vi "Pressure Temperature Monitor v2.vi"() -> ()   [LabVIEW 2016]
panel:
  in  "?":i32(ring)=1 items=["MKS 943 Cold Cathode"=1, "Thyracont All Range"=2]
  in  "?":i32(ring)=2 items=["MKS 943 Cold Cathode"=1, "Thyracont All Range"=2]
  in  "?":bool
  out "Pressure CH2":dbl=3.6243247155441205e-08 format="%#.2e"
  out "LL Pressure":dbl(graph)=3.6243247155441205e-08
  out "Tempreture CH2":dbl=27.062558993140346 format="%.1f"
  out "T2 Tempreture":dbl(graph)=27.062558993140346
  in  "Gain":dbl=-10.0 format="%#_13g"
  in  "Gain":dbl=-11.0 format="%#_13g"
  out "Tempreture CH1":dbl=400.77454527767986 format="%.1f"
  out "Pressure CH1":dbl=1.7126957385138226e-08 format="%#.2e"
  out "Heater Tempreture":dbl(graph)=400.77454527767986
  in  "?":bool
  out "Overdosing":bool
  in  "Dosing Limit":dbl=20.0 format="%#.2f"
  in  "Base Pressure":dbl=6.47 format="%#.2e"
  out "PRE Pressure":dbl(graph)=1.7126957385138226e-08
  out "L":dbl format="%.1f"
  in  "Pressure Limit":dbl=10.0 format="%#.2e"
  in  "?":bool
  # "LL Pressure (Torr)"
  # "PRE Pressure"
  # "Langmuir"
  # "(Torr)"
  # "(Torr)"
  # "CH1"
  # "CH2"
  # "Heater Temperature"
  # "T2"
  # "(°C )"
  # "(°C )"
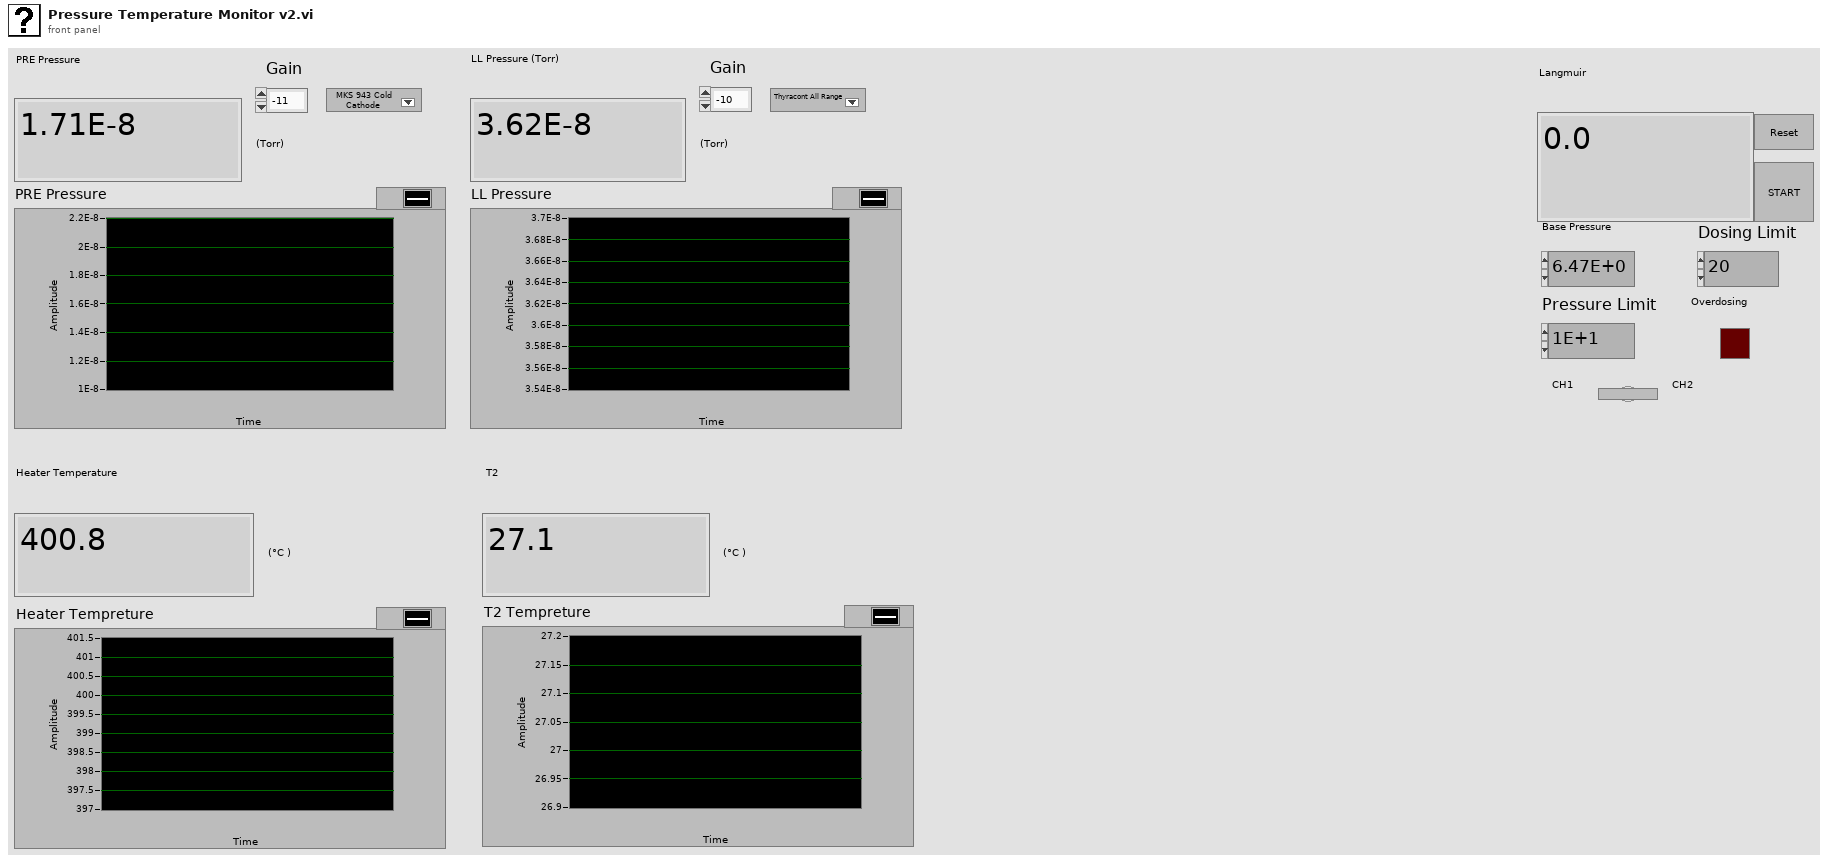
[diagram p1: front panel]
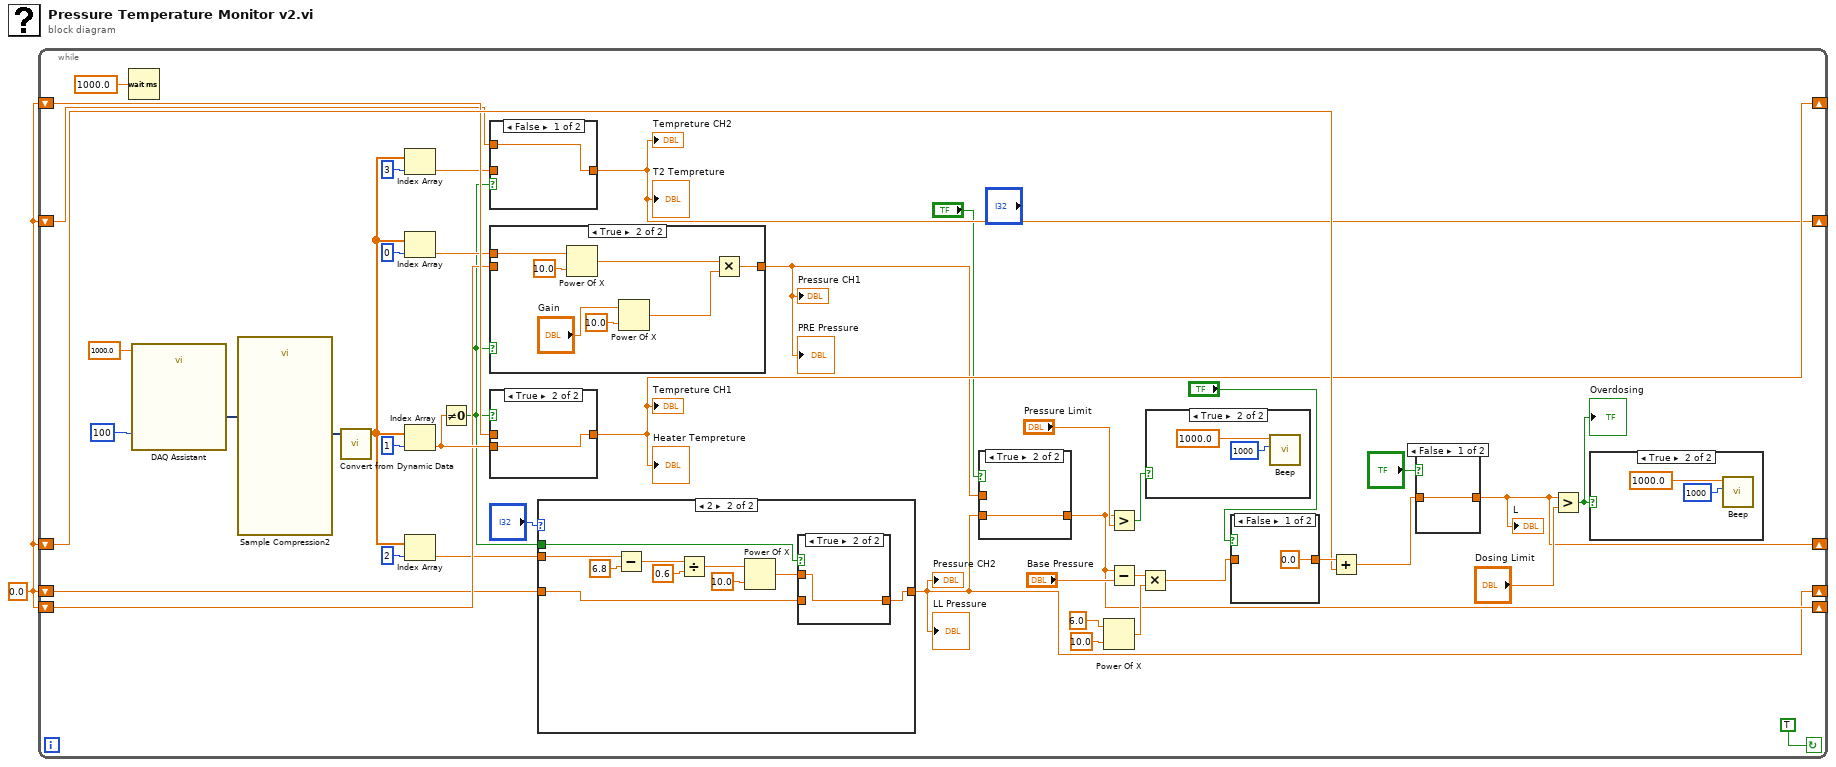
[diagram p0: block diagram]
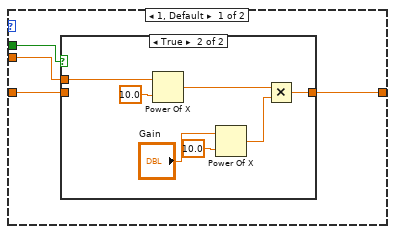
[diagram p2: hidden frame]
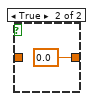
[diagram p9: hidden frame]
diagram:
  w1 = 0.0
  n1 = while {
    shift-left: w1 -> [w35]
    shift-right: [w33] -> _
    shift-right: [w6] -> _
    shift-left: w1 -> [w26]
    shift-right: [w25] -> _
    shift-left: w1 -> [w29]
    shift-right: [w4] -> _
    shift-left: w1 -> [w12]
    shift-right: [w9] -> _
    shift-left: w1 -> [w10]
    stop <- TRUE continue-if-true
    n2 = Wait (ms)(milliseconds to wait=1000.0 ("y")) -> ()  [unwired: 1 out]
    n3 = call "DAQ Assistant"("rate"=1000.0, "number of samples"=100) -> ("data"=w17:dynamicdata)  [unwired: 15 in, 2 out]
    n4 = call "Sample Compression2"("Signals"=w17) -> ("Mean"=w14:dynamicdata)  [unwired: 8 in, 2 out]
    n5 = call "Convert from Dynamic Data"("Dynamic Data Type"=w14) -> ("Array"=w3:dbl[])  [unwired: 3 in]
    n6 = Index Array(array=w3, index=3) -> (element=w11:dbl)
    n7 = Index Array(array=w3, index=0) -> (element=w27:dbl)
    n8 = Index Array(array=w3, index=1) -> (element=w28:dbl)
    n9 = Index Array(array=w3, index=2) -> (element=w13:dbl)
    n10 = Not Equal To 0?(x=w28) -> (x != 0?=w2:bool)
    n11 = case shown="False" w2 {
      tunnel: w10 -> [w71 _]
      tunnel: [w71 w72] -> w9
      tunnel: w11 -> [_ w72]
      frame False {
      }
      frame True {
      }
    }
    "T2 Tempreture" <- w9
    "Tempreture CH2" <- w9
    n12 = case shown="True" w2 {
      tunnel: w27 -> [_ w79]
      tunnel: [w73 w80] -> w7
      tunnel: w26 -> [w73 _]
      frame False {
      }
      frame True {
        n13 = Power Of X(1:10.0 ("x"), 2:w79) -> (0:w78:dbl)
        n14 = Power Of X(1:10.0 ("x"), 2:"Gain") -> (0:w76:dbl)
        n15 = Multiply(x=w78, y=w76) -> (x*y=w80:dbl)
      }
    }
    "PRE Pressure" <- w7
    "Pressure CH1" <- w7
    n16 = case shown="True" w2 {
      tunnel: w28 -> [_ w82]
      tunnel: [w81 w82] -> w25
      tunnel: w29 -> [w81 _]
      frame False {
      }
      frame True {
      }
    }
    "Heater Tempreture" <- w25
    "Tempreture CH1" <- w25
    n17 = case shown="2" "?" {
      tunnel: w2 -> [w48 w58]
      tunnel: w13 -> [w47 w57]
      tunnel: w12 -> [w46 w61]
      tunnel: [w45 w62] -> w4
      frame 1, Default {
        n18 = case shown="True" w48 {
          tunnel: w47 -> [_ w55]
          tunnel: [w49 w56] -> w45
          tunnel: w46 -> [w49 _]
          frame False {
          }
          frame True {
            n19 = Power Of X(1:10.0 ("x"), 2:w55) -> (0:w54:dbl)
            n20 = Power Of X(1:10.0 ("x"), 2:"Gain") -> (0:w52:dbl)
            n21 = Multiply(x=w54, y=w52) -> (x*y=w56:dbl)
          }
        }
      }
      frame 2 {
        n22 = Subtract(x=w57, y=6.8) -> (x-y=w64:dbl)
        n23 = Divide(x=w64, y=0.6) -> (x/y=w60:dbl)
        n24 = Power Of X(1:10.0 ("x"), 2:w60) -> (0:w59:dbl)
        n25 = case shown="True" w58 {
          tunnel: w59 -> [_ w68]
          tunnel: [w67 w68] -> w62
          tunnel: w61 -> [w67 _]
          frame False {
          }
          frame True {
          }
        }
      }
    }
    "LL Pressure" <- w4
    "Pressure CH2" <- w4
    n26 = case shown="True" "?" {
      tunnel: w7 -> [w69 _]
      tunnel: [w69 w70] -> w6
      tunnel: w4 -> [_ w70]
      frame False {
      }
      frame True {
      }
    }
    n27 = Power Of X(1:10.0 ("x"), 2:6.0 ("y")) -> (0:w21:dbl)
    n28 = Greater?(x=w6, y="Pressure Limit") -> (0:w43:bool)
    n29 = Subtract(x=w6, y="Base Pressure") -> (x-y=w24:dbl)
    n30 = Multiply(x=w24, y=w21) -> (x*y=w20:dbl)
    n31 = case shown="True" w43 {
      frame False {
      }
      frame True {
        n32 = call <vilib>:"Beep.vi"("duration (msec)"=i16 1000 ("duration (msec) - ignored"), "frequency (Hz)"=1000.0 ("frequency (Hz) - ignored")) -> ()  [unwired: 10 in]
      }
    }
    n33 = case shown="False" "?" {
      tunnel: [0.0 w88] -> w36
      tunnel: w20 -> [_ w88]
      frame False {
      }
      frame True {
      }
    }
    n34 = Add(x=w36, y=w35) -> (x+y=w34:dbl)
    n35 = case shown="False" "?" {
      tunnel: w34 -> [w83 _]
      tunnel: [w83 0.0 ("y")] -> w33
      frame False {
      }
      frame True {
      }
    }
    "L" <- w33
    n36 = Greater?(x=w33, y="Dosing Limit") -> (0:w37:bool)
    "Overdosing" <- w37
    n37 = case shown="True" w37 {
      frame False {
      }
      frame True {
        n38 = call <vilib>:"Beep.vi"("duration (msec)"=i16 1000 ("duration (msec) - ignored"), "frequency (Hz)"=1000.0 ("frequency (Hz) - ignored")) -> ()  [unwired: 10 in]
      }
    }
  }
